vi "GenerateArray.vi"() -> ()   [LabVIEW 2014]
panel:
  out "output array":dbl[](array[numeric])
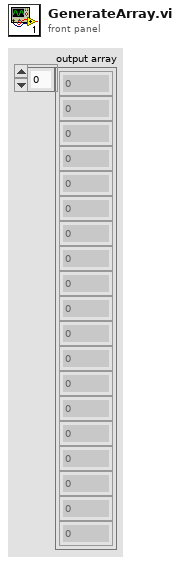
[diagram p1: front panel]
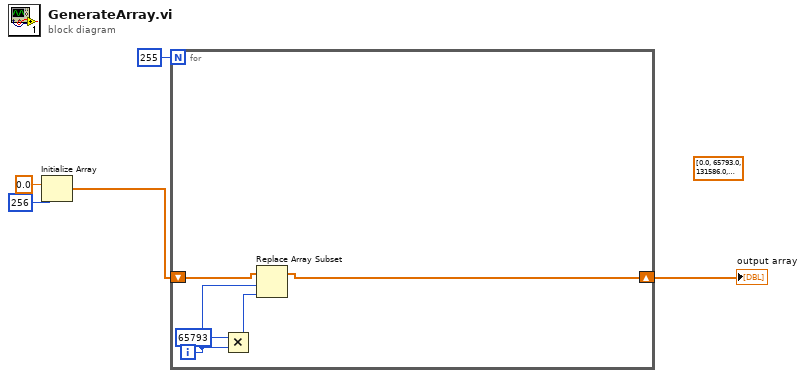
[diagram p0: block diagram]
diagram:
  (unwired) dbl[] [0.0, 65793.0, 131586.0, 197379.0, 263172.0, 328965.0, 394758.0, 460551.0, 526344.0, 592137.0, 657930.0, 723723.0, 789516.0, 855309.0, 921102.0, 986895.0, 1052688.0, 1118481.0, 1184274.0, 1250067.0, 1315860.0, 1381653.0, 1447446.0, 1513239.0, 1579032.0, 1644825.0, 1710618.0, 1776411.0, 1842204.0, 1907997.0, 1973790.0, 2039583.0, 2105376.0, 2171169.0, 2236962.0, 2302755.0, 2368548.0, 2434341.0, 2500134.0, 2565927.0, 2631720.0, 2697513.0, 2763306.0, 2829099.0, 2894892.0, 2960685.0, 3026478.0, 3092271.0, 3158064.0, 3223857.0, 3289650.0, 3355443.0, 3421236.0, 3487029.0, 3552822.0, 3618615.0, 3684408.0, 3750201.0, 3815994.0, 3881787.0, 3947580.0, 4013373.0, 4079166.0, 4144959.0, 4210752.0, 4276545.0, 4342338.0, 4408131.0, 4473924.0, 4539717.0, 4605510.0, 4671303.0, 4737096.0, 4802889.0, 4868682.0, 4934475.0, 5000268.0, 5066061.0, 5131854.0, 5197647.0, 5263440.0, 5329233.0, 5395026.0, 5460819.0, 5526612.0, 5592405.0, 5658198.0, 5723991.0, 5789784.0, 5855577.0, 5921370.0, 5987163.0, 6052956.0, 6118749.0, 6184542.0, 6250335.0, 6316128.0, 6381921.0, 6447714.0, 6513507.0, 6579300.0, 6645093.0, 6710886.0, 6776679.0, 6842472.0, 6908265.0, 6974058.0, 7039851.0, 7105644.0, 7171437.0, 7237230.0, 7303023.0, 7368816.0, 7434609.0, 7500402.0, 7566195.0, 7631988.0, 7697781.0, 7763574.0, 7829367.0, 7895160.0, 7960953.0, 8026746.0, 8092539.0, 8158332.0, 8224125.0, 8289918.0, 8355711.0, 8421504.0, 8487297.0, 8553090.0, 8618883.0, 8684676.0, 8750469.0, 8816262.0, 8882055.0, 8947848.0, 9013641.0, 9079434.0, 9145227.0, 9211020.0, 9276813.0, 9342606.0, 9408399.0, 9474192.0, 9539985.0, 9605778.0, 9671571.0, 9737364.0, 9803157.0, 9868950.0, 9934743.0, 10000536.0, 10066329.0, 10132122.0, 10197915.0, 10263708.0, 10329501.0, 10395294.0, 10461087.0, 10526880.0, 10592673.0, 10658466.0, 10724259.0, 10790052.0, 10855845.0, 10921638.0, 10987431.0, 11053224.0, 11119017.0, 11184810.0, 11250603.0, 11316396.0, 11382189.0, 11447982.0, 11513775.0, 11579568.0, 11645361.0, 11711154.0, 11776947.0, 11842740.0, 11908533.0, 11974326.0, 12040119.0, 12105912.0, 12171705.0, 12237498.0, 12303291.0, 12369084.0, 12434877.0, 12500670.0, 12566463.0, 12632256.0, 12698049.0, 12763842.0, 12829635.0, 12895428.0, 12961221.0, 13027014.0, 13092807.0, 13158600.0, 13224393.0, 13290186.0, 13355979.0, 13421772.0, 13487565.0, 13553358.0, 13619151.0, 13684944.0, 13750737.0, 13816530.0, 13882323.0, 13948116.0, 14013909.0, 14079702.0, 14145495.0, 14211288.0, 14277081.0, 14342874.0, 14408667.0, 14474460.0, 14540253.0, 14606046.0, 14671839.0, 14737632.0, 14803425.0, 14869218.0, 14935011.0, 15000804.0, 15066597.0, 15132390.0, 15198183.0, 15263976.0, 15329769.0, 15395562.0, 15461355.0, 15527148.0, 15592941.0, 15658734.0, 15724527.0, 15790320.0, 15856113.0, 15921906.0, 15987699.0, 16053492.0, 16119285.0, 16185078.0, 16250871.0, 16316664.0, 16382457.0, 16448250.0, 16514043.0, 16579836.0, 16645629.0, 16711422.0, 0.0] ("output array 2")
  n1 = Initialize Array(0.0 ("element"), 256 ("dimension size")) -> (w2:dbl[])
  n2 = for {
    N: 255 -> [_]
    shift-right: [w9] -> w1
    shift-left: w2 -> [w10]
    i -> [w8]
    n3 = Multiply(x=65793, y=w8) -> (x*y=w6:i32)
    n4 = Replace Array Subset(array=w10, new element=w6, index=w8) -> (w9:dbl[])
  }
  "output array" <- w1
